vi "Generate Gene.vi"(8 "error in":errorcluster, 10 "Gene Parameters":variant, 11 "Binary Gene in":refnum<class "Binary Gene.lvclass">) -> (0 "error out":errorcluster, 3 "Binary Gene out":refnum<class "Binary Gene.lvclass">)   [LabVIEW 2016, in "Binary Gene.lvclass"]
uses:
  Binary Gene.lvclass
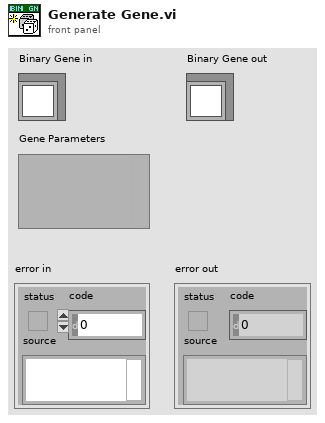
[diagram p1: front panel]
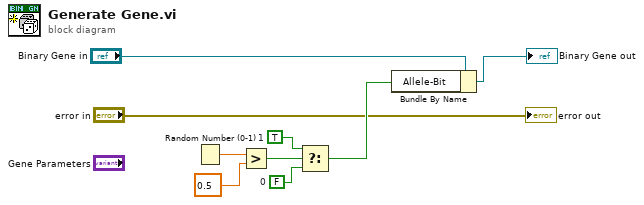
[diagram p0: block diagram]
diagram:
  w8 = TRUE  # 1
  w9 = FALSE  # 0
  n1 = Random Number (0-1)() -> (number: 0 to 1=w5:dbl)
  n2 = Greater?(x=w5, y=0.5) -> (0:w7:bool)
  n3 = Select(t=w8, s=w7, f=w9) -> (s? t:f=w2:bool)
  n4 = Bundle By Name(cluster="Binary Gene in", "Allele-Bit"=w2) -> (→"Binary Gene out":refnum<class "Binary Gene.lvclass">)
  "error out" <- "error in"
